vi "KE2260B Configure VI Level.vi"(8 "error in (no error)":errorcluster, 9 "Current Level (0.000 A)":dbl format="%.3g", 10 "Voltage Level (0.000 V)":dbl format="%.3g", 11 "VISA resource name":refnum<visa-resource-name>) -> (0 "error out":errorcluster, 3 "VISA resource name out":refnum<visa-resource-name>)   [LabVIEW 2021, in "Keithley 2260B.lvlib"]
doc: "Configures the output voltage level and the output current level."
uses:
  Keithley 2260B.lvlib
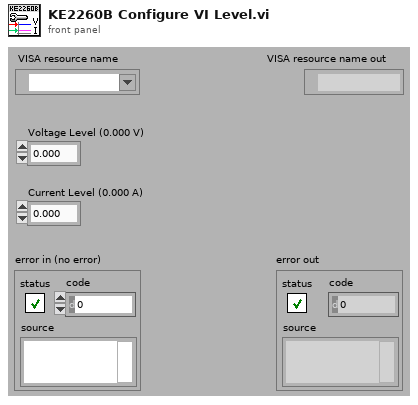
[diagram p1: front panel]
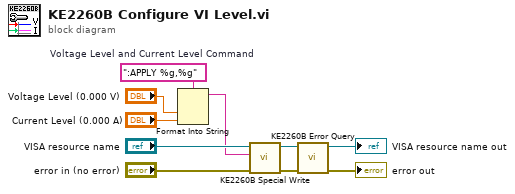
[diagram p0: block diagram]
diagram:
  w7 = ":APPLY %g,%g"  # Voltage Level and Current Level Command
  n1 = Format Into String(format string=w7, "Voltage Level (0.000 V)", "Current Level (0.000 A)") -> (resulting string=w2:string)  [unwired: 2 in, 1 out]
  n2 = call "KE2260B Special Write.vi"("error in (no error)"="error in (no error)", "Write Buffer (\"\")"=w2, "VISA session"="VISA resource name") -> ("error out"=w6:errorcluster, "dup VISA session"=w5:refnum<visa-resource-name>)  [unwired: 6 in, 1 out]
  n3 = call "KE2260B Error Query.vi"("error in (no error)"=w6, "VISA resource name"=w5) -> ("error out"=→"error out":errorcluster, "VISA resource name out"=→"VISA resource name out":refnum<visa-resource-name>)  [unwired: 6 in, 2 out]
